vi "Project Build Tools.vi"() -> (0 "Errors":errorcluster)   [LabVIEW 2019]
uses:
  Project Sync Tools/TypeDefs/Item Settings.ctl
  Project Build Tools/TypeDefs/Configure Build Types.ctl
  Project Sync Tools/TypeDefs/BuildSpec Source Parameters.ctl
  Project Sync Tools/TypeDefs/Source Parameters.ctl
  Project Sync Tools/Project Sync Tools.lvclass/Project Sync Tools.ctl
  Project Build Tools/Project Build Tools.lvclass/Project Build Tools.ctl
  Project Build Tools/Project Build Tools.lvclass
  Project XML Editor/Project XML Editor.lvclass
  Project Sync Tools/Project Sync Tools.lvclass
panel:
  in  "Perform Project Clean-up?":bool
  out "Progress Status":string
  in  "Project Path":path
  out "Build Progress":u8(slide) scale=0.0..100.0
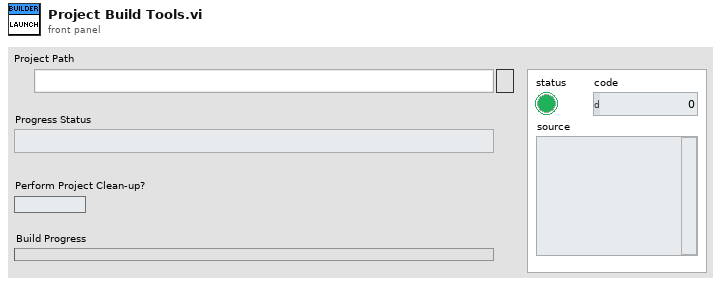
[diagram p1: front panel]
types:
  T1 = typedef "Project Sync Tools.lvclass/BuildSpec Source Parameters.ctl" = cluster{"BuildSpec Name":string, "Sources":T2[]}
  T2 = typedef "Project Sync Tools.lvclass/Source Parameters.ctl" = cluster{"Source Library":string, "Source Item Name":string, "Destination Label":string, "Item Type":string, "Apply Inclusion":bool}
  T3 = typedef "Project Build Tools.lvclass/Configure Build Types.ctl" = enum16{"DLL", "Packed Library", "Installer", "Source Distribution", "EXE"}
  T4 = typedef "Project Sync Tools.lvclass/Item Settings.ctl" = cluster{"Item Name":string, "Item Type":string, "Item Parameters":variant}
  T5 = typedef "Project XML Editor.lvclass/Dependency Parameters.ctl" = cluster{"Supported Target":string, "RT System Destination":string, "Source Path (Relative)":string}
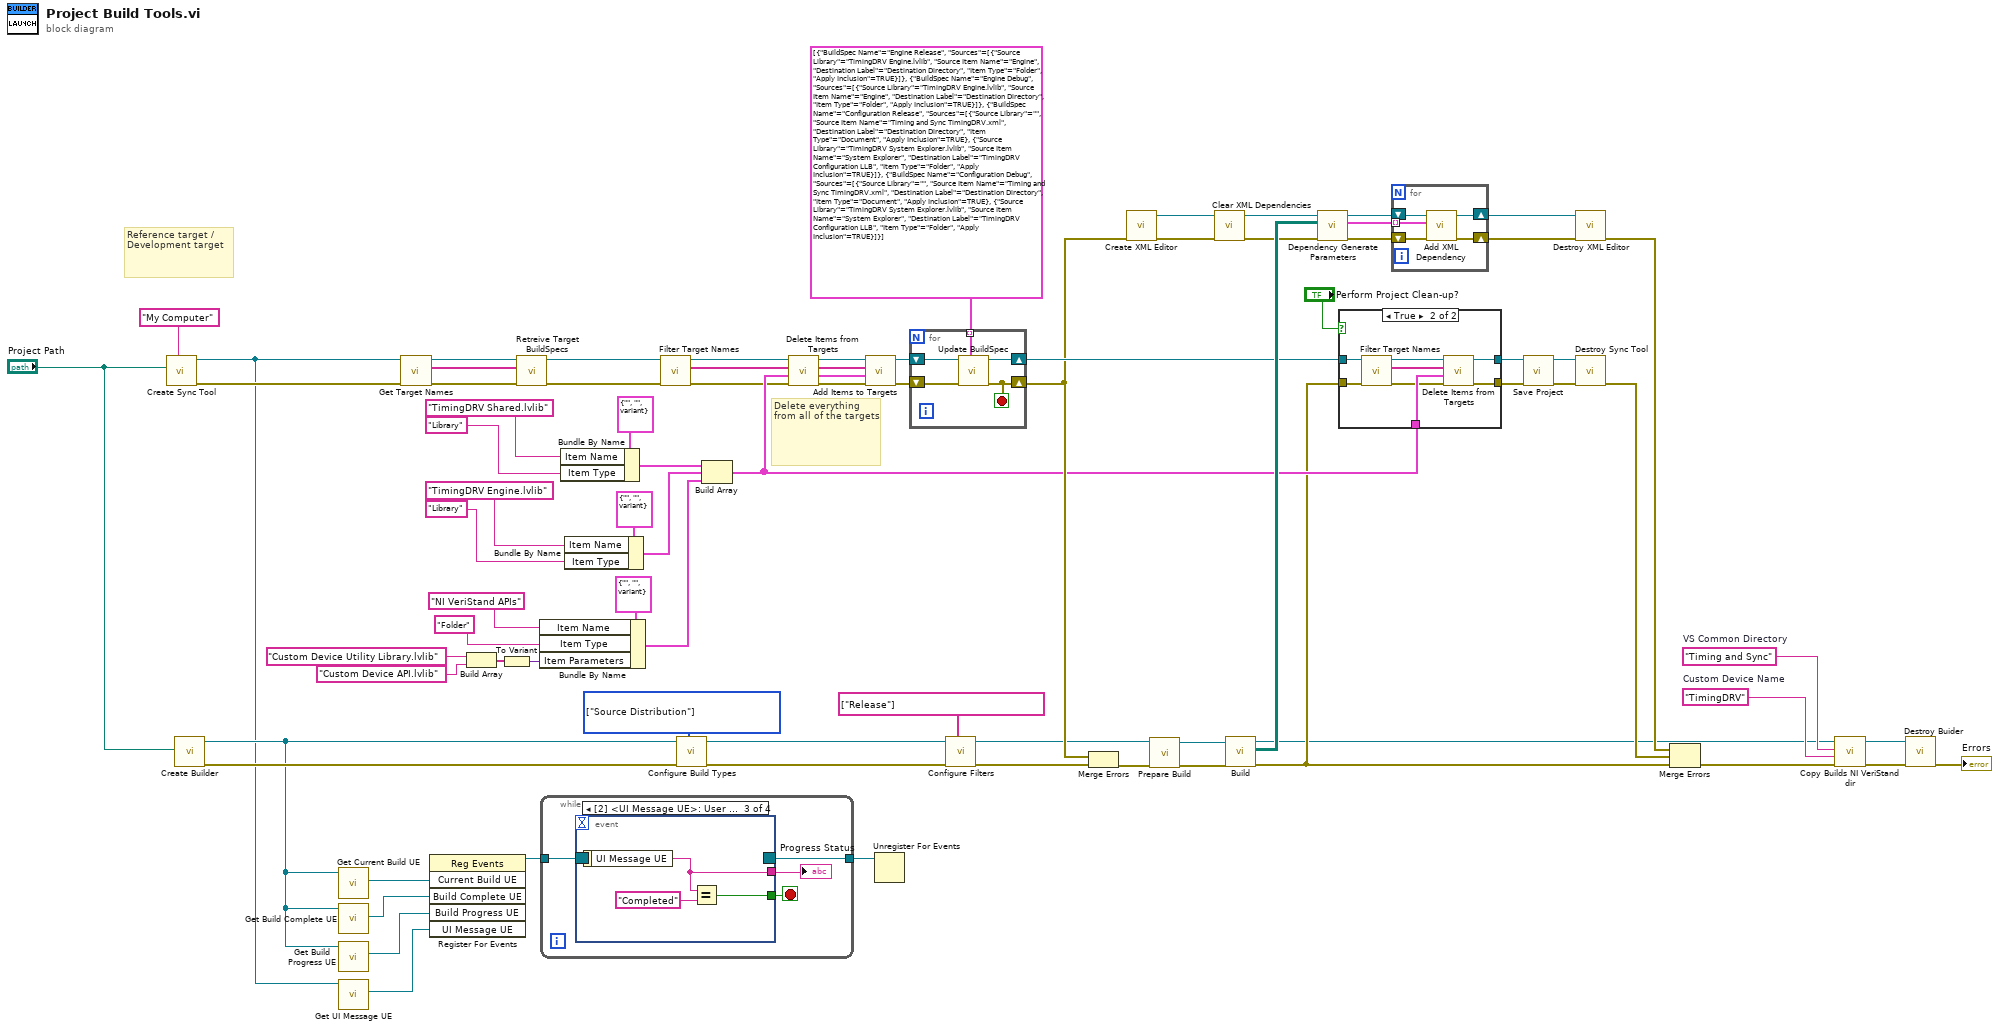
[diagram p0: block diagram]
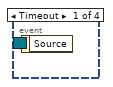
[diagram p3: hidden frame]
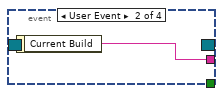
[diagram p4: hidden frame]
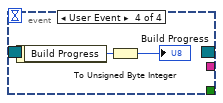
[diagram p5: hidden frame]
diagram:
  w17 = "TimingDRV"  # Custom Device Name
  w18 = "Timing and Sync"  # VS Common Directory
  w28 = T3[] [enum."Source Distribution"] items=["DLL", "Packed Library", "Installer", "Source Distribution", "EXE"] ("Build Types")
  # "Reference target / Development target"
  # "Delete everything from all of the targets"
  n1 = call "Create Sync Tool.vi"("Reference Target Name"="My Computer" ("Target Name"), "Project Path"="Project Path") -> ("error out"=w12:errorcluster, "CD Build Tools out"=w2:refnum<class "Project Sync Tools.lvclass">)  [unwired: 8 in]
  n2 = call "Create Builder.vi"("File Path Control"="Project Path") -> ("error out"=w27:errorcluster, "CD Build Tools out"=w26:refnum<class "Project Build Tools.lvclass">)  [unwired: 9 in]
  n3 = call "Get Current Build UE.vi"("CD Build Tools in"=w26) -> ("Current Build UE"=w80:refnum<user-event>)  [unwired: 9 in, 1 out]
  n4 = call "Get Build Complete UE.vi"("CD Build Tools in"=w26) -> ("Build Complete UE"=w78:refnum<user-event>)  [unwired: 9 in, 1 out]
  n5 = call "Get Build Progress UE.vi"("CD Build Tools in"=w26) -> ("Build Progress UE"=w76:refnum<user-event>)  [unwired: 9 in, 1 out]
  n6 = call "Get UI Message UE.vi"("Project Sync Tools in"=w2) -> ("UI Message UE"=w36:refnum<user-event>)  [unwired: 9 in, 1 out]
  n7 = call "Get Target Names.vi"("error in (no error)"=w12, "Project Sync Tools in"=w2) -> ("error out"=w9:errorcluster, "Targets names"=w10:string[], "Project Sync Tools out"=w11:refnum<class "Project Sync Tools.lvclass">)  [unwired: 7 in]
  n8 = register-events(w80, w78, w76, w36) -> (reference out=w79:refnum<event-registration>)  [unwired: 2 in, 1 out]
  n9 = Build Array("Custom Device Utility Library.lvlib" ("Library Name"), "Custom Device API.lvlib" ("Library Name")) -> (w49:string[])
  n10 = To Variant(anything=w49) -> (Variant=w48:variant)
  n11 = call "Retreive Target BuildSpecs.vi"("error in (no error)"=w9, "Target Names in"=w10, "Project Sync Tools in"=w11) -> ("error out"=w5:errorcluster, "Project Sync Tools out"=w4:refnum<class "Project Sync Tools.lvclass">)  [unwired: 6 in, 1 out]
  n12 = Bundle By Name(cluster=T4 {"Item Name"="", "Item Type"="", "Item Parameters"=variant}, "Item Name"="NI VeriStand APIs" ("Name"), "Item Type"="Folder", "Item Parameters"=w48) -> (w46:T4)
  n13 = while {
    tunnel: w79 -> [w84]
    tunnel: [w82] -> w77
    stop <- w83 stop-if-true
    n14 = event shown="[2] <UI Message UE>: User Event" {
      selector: w84 -> [_ _ _ _]
      dyn-events: [_ _ _ _] -> w82
      timeout: _ -> [_ _ _ _]
      tunnel: [_ _ w87 _] -> w83
      tunnel: [_ w85 w86 _] -> w81
      event Timeout {
        n15 = event-data() -> ()  [unwired: 1 in, 1 out]
      }
      event User Event {
        n16 = event-data() -> ("Current Build"=w85:string)  [unwired: 1 in]
      }
      event User Event {
        n17 = event-data() -> ("UI Message UE"=w86:string)  [unwired: 1 in]
        n18 = Equal?(x=w86, y="Completed") -> (x = y?=w87:bool)
      }
      event User Event {
        n19 = event-data() -> ("Build Progress"=w90:i32)  [unwired: 1 in]
        n20 = To Unsigned Byte Integer(number=w90) -> (unsigned 8bit integer=→"Build Progress":u8)
      }
    }
    "Progress Status" <- w81
  }
  n21 = Bundle By Name(cluster=T4 {"Item Name"="", "Item Type"="", "Item Parameters"=variant}, "Item Name"="TimingDRV Shared.lvlib", "Item Type"="Library") -> (w60:T4)
  n22 = Bundle By Name(cluster=T4 {"Item Name"="", "Item Type"="", "Item Parameters"=variant}, "Item Name"="TimingDRV Engine.lvlib" ("Library Name"), "Item Type"="Library") -> (w54:T4)
  n23 = call "Filter Target Names.vi"("error in (no error)"=w5, "Project Sync Tools in"=w4) -> ("error out"=w7:errorcluster, "Filtered Names"=w6:string[], "Project Sync Tools out"=w8:refnum<class "Project Sync Tools.lvclass">)  [unwired: 7 in]
  n24 = call "Configure Build Types.vi"("Build Types"=w28, "error in (no error)"=w27, "CD Build Tools in"=w26) -> ("error out"=w31:errorcluster, "CD Build Tools out"=w30:refnum<class "Project Build Tools.lvclass">)  [unwired: 7 in]
  n25 = Build Array(w60, w54, w46) -> (w32:T4[])
  n26 = call "Delete Items from Targets.vi"("error in (no error)"=w7, "Items"=w32, "Targets in"=w6, "Project Sync Tools in"=w8) -> ("error out"=w41:errorcluster, "Items out"=w40:T4[], "Targets out"=w42:string[], "Project Sync Tools out"=w43:refnum<class "Project Sync Tools.lvclass">)  [unwired: 4 in]
  n27 = call "Add Items to Targets.vi"("error in (no error)"=w41, "Items in"=w40, "Target Names in"=w42, "Project Sync Tools in"=w43) -> ("error out"=w44:errorcluster, "Project Sync Tools out"=w45:refnum<class "Project Sync Tools.lvclass">)  [unwired: 4 in, 2 out]
  n28 = Unregister For Events(event registration refnum=w77) -> ()  [unwired: 1 in, 1 out]
  n29 = for {
    shift-right: [w95] -> w39
    shift-left: w45 -> [w94]
    shift-right: [w91] -> w33
    shift-left: w44 -> [w93]
    tunnel: T1[] [{"BuildSpec Name"="Engine Release", "Sources"=[{"Source Library"="TimingDRV Engine.lvlib", "Source Item Name"="Engine", "Destination Label"="Destination Directory", "Item Type"="Folder", "Apply Inclusion"=TRUE}]}, {"BuildSpec Name"="Engine Debug", "Sources"=[{"Source Library"="TimingDRV Engine.lvlib", "Source Item Name"="Engine", "Destination Label"="Destination Directory", "Item Type"="Folder", "Apply Inclusion"=TRUE}]}, {"BuildSpec Name"="Configuration Release", "Sources"=[{"Source Library"="", "Source Item Name"="Timing and Sync TimingDRV.xml", "Destination Label"="Destination Directory", "Item Type"="Document", "Apply Inclusion"=TRUE}, {"Source Library"="TimingDRV System Explorer.lvlib", "Source Item Name"="System Explorer", "Destination Label"="TimingDRV Configuration LLB", "Item Type"="Folder", "Apply Inclusion"=TRUE}]}, {"BuildSpec Name"="Configuration Debug", "Sources"=[{"Source Library"="", "Source Item Name"="Timing and Sync TimingDRV.xml", "Destination Label"="Destination Directory", "Item Type"="Document", "Apply Inclusion"=TRUE}, {"Source Library"="TimingDRV System Explorer.lvlib", "Source Item Name"="System Explorer", "Destination Label"="TimingDRV Configuration LLB", "Item Type"="Folder", "Apply Inclusion"=TRUE}]}] -> [w92] mode=indexing
    stop <- w91 stop-if-true
    n30 = call "Update BuildSpec.vi"("Buildspec Source Parameters"=w92, "error in (no error)"=w93, "CD Build Tools in"=w94) -> ("error out"=w91:errorcluster, "CD Build Tools out"=w95:refnum<class "Project Sync Tools.lvclass">)  [unwired: 7 in]
  }
  n31 = call "Configure Filters.vi"("Name Filters"=string[] ["Release"] ("Filters"), "error in (no error)"=w31, "CD Build Tools in"=w30) -> ("error out"=w25:errorcluster, "CD Build Tools out"=w24:refnum<class "Project Build Tools.lvclass">)  [unwired: 7 in]
  n32 = Merge Errors(w33, w25) -> (w23:errorcluster)
  n33 = call "Create XML Editor.vi"("error in (no error)"=w33) -> ("error out"=w72:errorcluster, "Project XML Editor out"=w73:refnum<class "Project XML Editor.lvclass">)  [unwired: 9 in]
  n34 = call "Prepare Build.vi"("error in (no error)"=w23, "CD Build Tools in"=w24) -> ("error out"=w21:errorcluster, "CD Build Tools out"=w22:refnum<class "Project Build Tools.lvclass">)  [unwired: 8 in]
  n35 = call "Clear XML Dependencies.vi"("error in (no error)"=w72, "Project XML Editor in"=w73) -> ("error out"=w66:errorcluster, "Project XML Editor out"=w71:refnum<class "Project XML Editor.lvclass">)  [unwired: 8 in]
  n36 = call "Build.vi"("error in (no error)"=w21, "CD Build Tools in"=w22) -> ("error out"=w16:errorcluster, "Generated files"=w67:path[][], "CD Build Tools out"=w13:refnum<class "Project Build Tools.lvclass">)  [unwired: 7 in]
  n37 = call "Dependency Generate Parameters.vi"("error in (no error)"=w66, "Generated files in"=w67, "Project XML Editor in"=w71) -> ("error out"=w70:errorcluster, "Dependency Parameters"=w68:T5[], "Project XML Editor out"=w69:refnum<class "Project XML Editor.lvclass">)  [unwired: 6 in]
  n38 = case shown="True" "Perform Project Clean-up?" {
    tunnel: w16 -> [w96 w105]
    tunnel: w39 -> [w97 w104]
    tunnel: [w96 w103] -> w63
    tunnel: [w97 w102] -> w62
    tunnel: w32 -> [_ w101]
    frame False {
    }
    frame True {
      n39 = call "Filter Target Names.vi"("error in (no error)"=w105, "Project Sync Tools in"=w104) -> ("error out"=w98:errorcluster, "Filtered Names"=w99:string[], "Project Sync Tools out"=w100:refnum<class "Project Sync Tools.lvclass">)  [unwired: 7 in]
      n40 = call "Delete Items from Targets.vi"("error in (no error)"=w98, "Items"=w101, "Targets in"=w99, "Project Sync Tools in"=w100) -> ("error out"=w103:errorcluster, "Project Sync Tools out"=w102:refnum<class "Project Sync Tools.lvclass">)  [unwired: 4 in, 2 out]
    }
  }
  n41 = for {
    shift-right: [w109] -> w74
    shift-left: w70 -> [w108]
    shift-right: [w110] -> w75
    shift-left: w69 -> [w107]
    tunnel: w68 -> [w106] mode=indexing
    n42 = call "Add XML Dependency.vi"("error in (no error)"=w108, "Dependency Parameters"=w106, "Project XML Editor in"=w107) -> ("error out"=w109:errorcluster, "Project XML Editor out"=w110:refnum<class "Project XML Editor.lvclass">)  [unwired: 7 in]
  }
  n43 = call "Save Project.vi"("error in (no error)"=w63, "Project Sync Tools in"=w62) -> ("error out"=w65:errorcluster, "Project Sync Tools out"=w64:refnum<class "Project Sync Tools.lvclass">)  [unwired: 8 in]
  n44 = call "Destroy XML Editor.vi"("error in (no error)"=w74, "Project XML Editor in"=w75) -> ("error out"=w38:errorcluster)  [unwired: 9 in]
  n45 = call "Destroy Sync Tool.vi"("error in (no error)"=w65, "CD Build Tools in"=w64) -> ("error out"=w37:errorcluster)  [unwired: 9 in]
  n46 = Merge Errors(w38, w37, w16) -> (w15:errorcluster)
  n47 = call "Copy Builds NI VeriStand dir.vi"("error in (no error)"=w15, "Custom Device Name"=w17, "VS Common Directory"=w18, "CD Build Tools in"=w13) -> ("error out"=w19:errorcluster, "CD Build Tools out"=w20:refnum<class "Project Build Tools.lvclass">)  [unwired: 6 in]
  n48 = call "Destroy Buider.vi"("error in (no error)"=w19, "CD Build Tools in"=w20) -> ("error out"=→"Errors":errorcluster)  [unwired: 9 in]
